vi "set galvo trigger.vi"(8 "error in (no error)":errorcluster, 11 "Waveform in":refnum<class "Waveform.lvclass">) -> (0 "error out":errorcluster, 3 "Waveform out":refnum<class "Waveform.lvclass">)   [LabVIEW 2012, in "Waveform.lvclass"]
uses:
  Waveform.lvclass
  Waveform.lvclass/Waveform.ctl
  <vilib>/DAQmx/configure/trigger.llb/DAQmx Start Trigger (Digital Edge).vi
  <resource>/objmgr/daqmx.rc
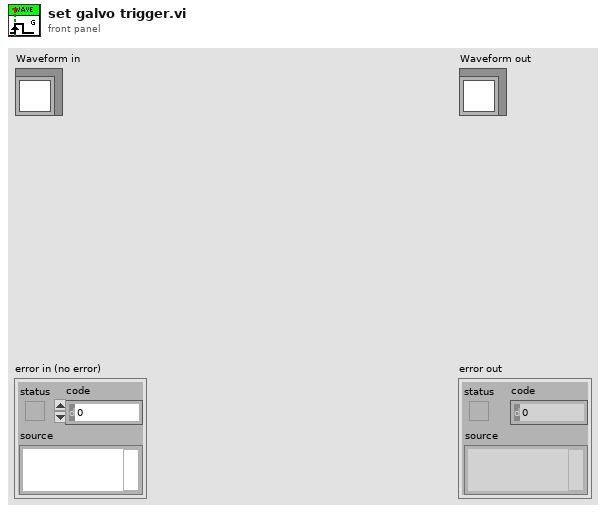
[diagram p1: front panel]
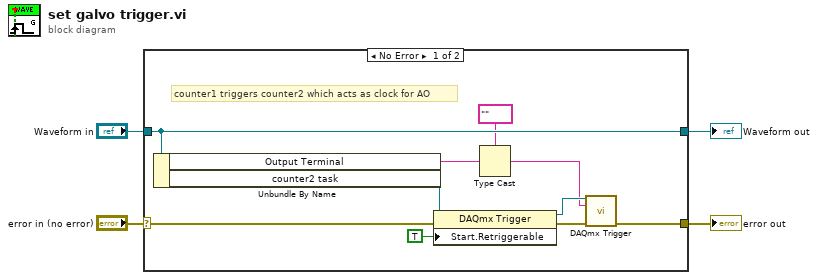
[diagram p0: block diagram]
diagram:
  n1 = case shown="No Error" "error in (no error)" {
    selector: "error in (no error)" -> [w14 w16]
    tunnel: [w6 w16] -> w3
    tunnel: [w10 w15] -> w1
    tunnel: "Waveform in" -> [w10 w15]
    frame No Error {
      # "counter1 triggers counter2 which acts as clock for AO"
      n2 = Unbundle By Name(w10) -> ("Output Terminal"=w9:string, "counter2 task"=w11:refnum<k21>)
      n3 = property class="DAQmx Trigger"(reference=w11, error in=w14, "Start.Retriggerable"=TRUE) -> (reference out=w7:refnum<k21>, error out=w12:errorcluster)
      n4 = Type Cast(type=tag "" ("source"), x=w9) -> (*(type *) &x=w5:tag)
      n5 = call-poly <vilib>:"DAQmx Trigger.vi"("task/channels in"=w7, "source"=w5, "error in"=w12) -> ("error out"=w6:errorcluster)  [unwired: 11 in, 1 out]
    }
    frame Error {
    }
  }
  "error out" <- w3
  "Waveform out" <- w1
